vi "pump_main.vi"(8 "error in (no error)":errorcluster, 10 "input string":string, 11 "VISA resource name":refnum<visa-resource-name>) -> (0 "error out":errorcluster, 3 "VISA resource name out":refnum<visa-resource-name>)   [LabVIEW 2020]
uses:
  status/emergency stop.vi
panel:
  out "current time 2":timestamp
  out "current time":timestamp
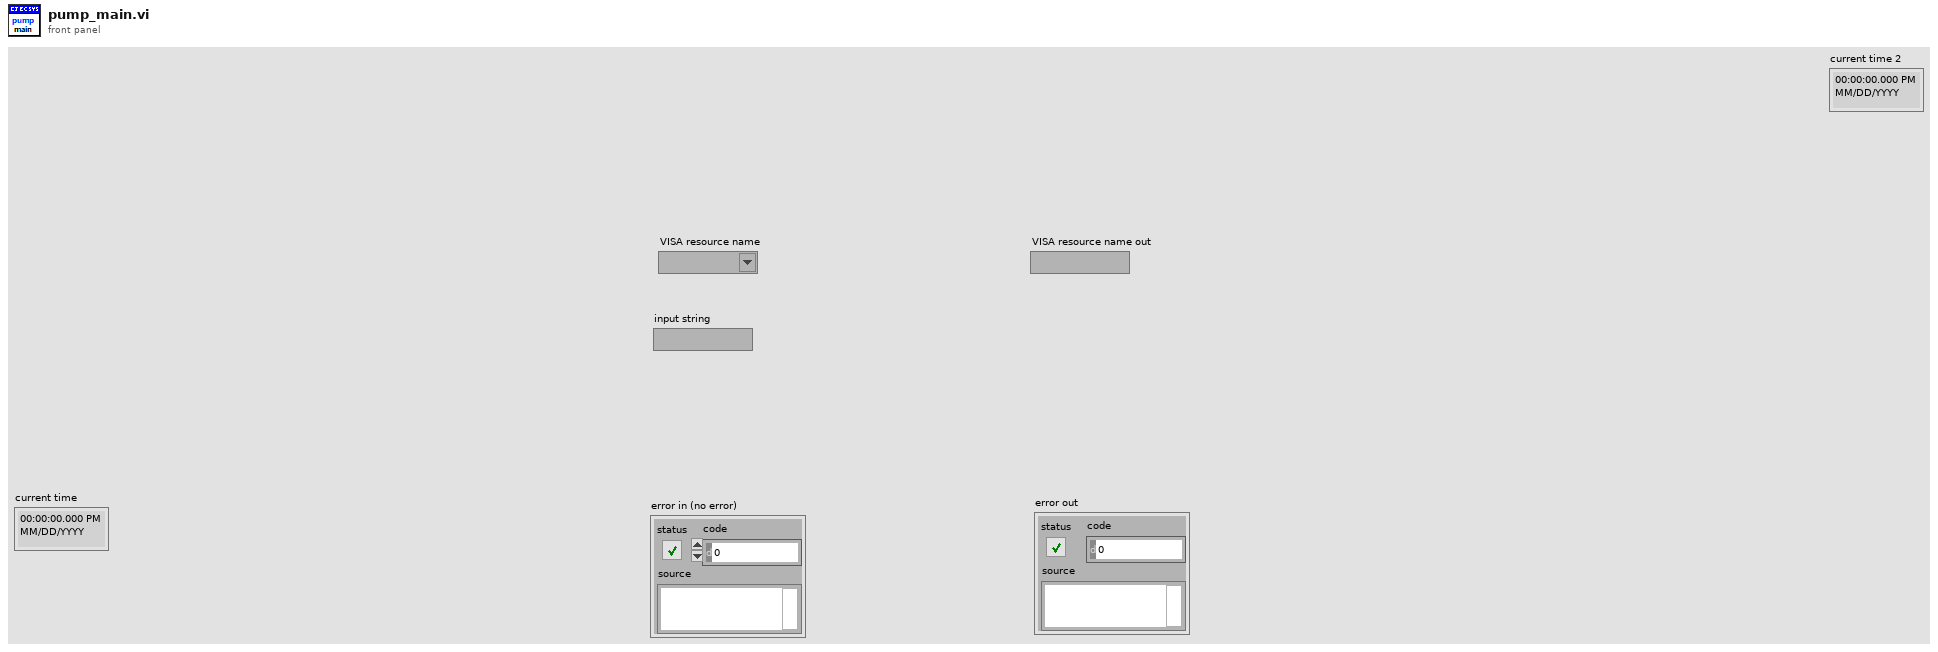
[diagram p1: front panel]
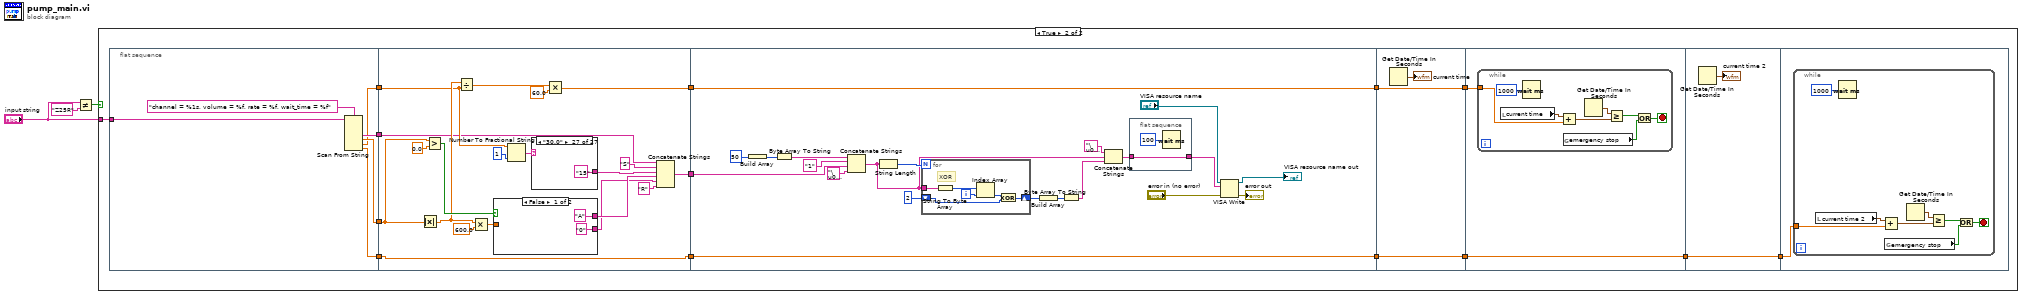
[diagram p0: block diagram]
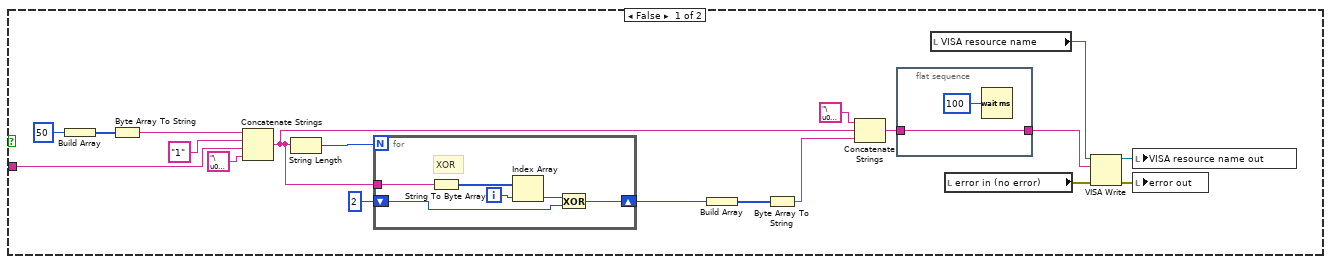
[diagram p2: hidden frame]
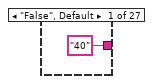
[diagram p3: hidden frame]
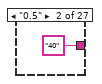
[diagram p4: hidden frame]
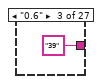
[diagram p5: hidden frame]
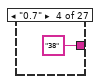
[diagram p6: hidden frame]
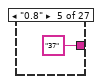
[diagram p7: hidden frame]
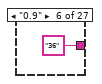
[diagram p8: hidden frame]
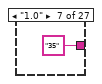
[diagram p9: hidden frame]
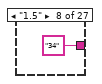
[diagram p10: hidden frame]
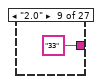
[diagram p11: hidden frame]
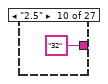
[diagram p12: hidden frame]
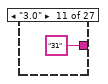
[diagram p13: hidden frame]
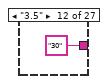
[diagram p14: hidden frame]
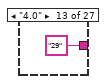
[diagram p15: hidden frame]
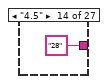
[diagram p16: hidden frame]
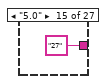
[diagram p17: hidden frame]
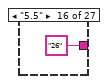
[diagram p18: hidden frame]
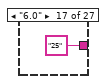
[diagram p19: hidden frame]
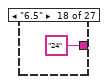
[diagram p20: hidden frame]
diagram:
  n1 = Not Equal?(x="input string", y="Z25R") -> (x != y?=w1:bool)
  n2 = case shown="True" w1 {
    tunnel: "input string" -> [w4 w31]
    frame False {
      n3 = Build Array(u8 50 ("y")) -> (w12:u8[])
      n4 = Byte Array To String(unsigned byte array=w12) -> (string=w10:string)
      n5 = Concatenate Strings(w10, "1" ("string"), w4, "\u0003" ("string")) -> (w16:string)
      n6 = String Length(string=w16) -> (length=w22:i32)
      n7 = for {
        N: w22 -> [_]
        tunnel: w16 -> [w30]
        shift-right: [w25] -> w20
        shift-left: u8 2 -> [w26]
        i -> [w28]
        # "XOR"
        n8 = String To Byte Array(string=w30) -> (unsigned byte array=w29:u8[])
        n9 = Index Array(array=w29, index=w28) -> (element=w27:u8)
        n10 = Exclusive Or(1:w26, 2:w27) -> (0:w25:u8)
      }
      n11 = Build Array(w20) -> (w19:u8[])
      n12 = Byte Array To String(unsigned byte array=w19) -> (string=w17:string)
      n13 = Concatenate Strings("\u0002" ("string"), w16, w17) -> (w15:string)
      n14 = flat-sequence {
        tunnel: [w24] -> w14
        tunnel: w15 -> [w24]
        frame #0 {
          n15 = Wait (ms)(milliseconds to wait=u32 100) -> ()  [unwired: 1 out]
        }
      }
      n16 = local read "VISA resource name"() -> (w8:refnum<visa-resource-name>)
      n17 = local read "error in (no error)"() -> (w7:errorcluster)
      n18 = VISA Write(VISA resource name=w8, write buffer=w14, error in (no error)=w7) -> (VISA resource name out=w6:refnum<visa-resource-name>, error out=w5:errorcluster)  [unwired: 1 out]
      n19 = local write "VISA resource name out"(w6) -> ()
      n20 = local write "error out"(w5) -> ()
    }
    frame True {
      n21 = flat-sequence {
        tunnel: [w49] -> w44
        tunnel: [w48] -> w43
        tunnel: [w47] -> w42
        tunnel: [w46] -> w41
        tunnel: w31 -> [w45]
        tunnel: [w66] -> w40
        tunnel: [w59] -> w39
        tunnel: w44 -> [w53]
        tunnel: w43 -> [w58]
        tunnel: w42 -> [w57]
        tunnel: w41 -> [w56]
        tunnel: [w56] -> w38
        tunnel: w40 -> [w109]
        tunnel: w39 -> [w104]
        tunnel: [w104] -> w37
        tunnel: w38 -> [w103]
        tunnel: [w103] -> w36
        tunnel: w37 -> [w133]
        tunnel: [w133] -> w35
        tunnel: [w132] -> w34
        tunnel: w36 -> [w132]
        tunnel: w35 -> [w136]
        tunnel: w34 -> [w135]
        tunnel: [w135] -> w33
        tunnel: w33 -> [w145]
        tunnel: [w145] -> w32
        tunnel: w32 -> [w147]
        frame #0 {
          n22 = Scan From String(format string="channel = %1s, volume = %f, rate = %f, wait_time = %f", input string=w45) -> (output 1=w49:string, output 2=w48:dbl, output 3=w47:dbl, output 4=w46:dbl)  [unwired: 6 in, 3 out]
        }
        frame #1 {
          n23 = Absolute Value(x=w58) -> (abs(x)=w62:dbl)
          n24 = Greater?(x=w58, y=0.0) -> (0:w69:bool)
          n25 = Divide(x=w62, y=w57) -> (x/y=w61:dbl)
          n26 = Multiply(x=w62, y=600.0) -> (x*y=w52:dbl)
          n27 = case shown="False" w69 {
            tunnel: ["A" ("channel") "P" ("channel")] -> w70
            tunnel: w52 -> [_ w101]
            tunnel: ["0" w100] -> w51
            frame False {
            }
            frame True {
              n28 = Number To Decimal String(number=w101) -> (decimal integer string=w100:string)  [unwired: 1 in]
            }
          }
          n29 = Number To Fractional String(number=w57, precision (6)=i16 1) -> (F-format string=w65:string)  [unwired: 2 in]
          n30 = case shown="\"30.0\"" w65 {
            tunnel: ["40" "40" "39" "38" "37" "36" "35" "34" "33" "32" "31" "30" "29" "28" "27" "26" "25" "24" "23" "22" "21" "20" "19" "18" "17" "16" "15"] -> w55
            frame "False", Default {
            }
            frame "0.5" {
            }
            frame "0.6" {
            }
            frame "0.7" {
            }
            frame "0.8" {
            }
            frame "0.9" {
            }
            frame "1.0" {
            }
            frame "1.5" {
            }
            frame "2.0" {
            }
            frame "2.5" {
            }
            frame "3.0" {
            }
            frame "3.5" {
            }
            frame "4.0" {
            }
            frame "4.5" {
            }
            frame "5.0" {
            }
            frame "5.5" {
            }
            frame "6.0" {
            }
            frame "6.5" {
            }
            frame "7.0" {
            }
            frame "7.5" {
            }
            frame "8.0" {
            }
            frame "8.5" {
            }
            frame "9.0" {
            }
            frame "9.5" {
            }
            frame "10.0" {
            }
            frame "20.0" {
            }
            frame "30.0" {
            }
          }
          n31 = Multiply(x=w61, y=60.0) -> (x*y=w59:dbl)
          n32 = Concatenate Strings(w53, "S" ("string"), w55, w70, w51, "R" ("string")) -> (w66:string)
        }
        frame #2 {
          n33 = Build Array(u8 50 ("y")) -> (w108:u8[])
          n34 = Byte Array To String(unsigned byte array=w108) -> (string=w106:string)
          n35 = Concatenate Strings(w106, "1" ("string"), w109, "\u0003" ("string")) -> (w117:string)
          n36 = String Length(string=w117) -> (length=w123:i32)
          n37 = for {
            N: w123 -> [_]
            tunnel: w117 -> [w131]
            shift-right: [w126] -> w121
            shift-left: u8 2 -> [w127]
            i -> [w129]
            # "XOR"
            n38 = String To Byte Array(string=w131) -> (unsigned byte array=w130:u8[])
            n39 = Index Array(array=w130, index=w129) -> (element=w128:u8)
            n40 = Exclusive Or(1:w127, 2:w128) -> (0:w126:u8)
          }
          n41 = Build Array(w121) -> (w120:u8[])
          n42 = Byte Array To String(unsigned byte array=w120) -> (string=w118:string)
          n43 = Concatenate Strings("\u0002" ("string"), w117, w118) -> (w114:string)
          n44 = flat-sequence {
            tunnel: [w125] -> w113
            tunnel: w114 -> [w125]
            frame #0 {
              n45 = Wait (ms)(milliseconds to wait=u32 100) -> ()  [unwired: 1 out]
            }
          }
          n46 = VISA Write(VISA resource name="VISA resource name", write buffer=w113, error in (no error)="error in (no error)") -> (VISA resource name out=→"VISA resource name out":refnum<visa-resource-name>, error out=→"error out":errorcluster)  [unwired: 1 out]
        }
        frame #3 {
          n47 = Get Date/Time In Seconds() -> (seconds since 1Jan1904=→"current time":timestamp)
        }
        frame #4 {
          n48 = while {
            tunnel: w136 -> [w138]
            stop <- w139 stop-if-true
            n49 = local read "current time"() -> (w143:timestamp)
            n50 = Wait (ms)(milliseconds to wait=u32 1000 ("millisecond timer value")) -> ()  [unwired: 1 out]
            n51 = Add(x=w143, y=w138) -> (x+y=w142:timestamp)
            n52 = global read "emergency stop.vi" "emergency stop"() -> (w137:bool)
            n53 = Get Date/Time In Seconds() -> (seconds since 1Jan1904=w141:timestamp)
            n54 = Greater Or Equal?(x=w141, y=w142) -> (x >= y?=w140:bool)
            n55 = Or(x=w140, y=w137) -> (x .or. y?=w139:bool)
          }
        }
        frame #5 {
          n56 = Get Date/Time In Seconds() -> (seconds since 1Jan1904=→"current time 2":timestamp)
        }
        frame #6 {
          n57 = while {
            tunnel: w147 -> [w149]
            stop <- w150 stop-if-true
            n58 = local read "current time 2"() -> (w154:timestamp)
            n59 = Wait (ms)(milliseconds to wait=u32 1000 ("millisecond timer value")) -> ()  [unwired: 1 out]
            n60 = Add(x=w154, y=w149) -> (x+y=w153:timestamp)
            n61 = global read "emergency stop.vi" "emergency stop"() -> (w148:bool)
            n62 = Get Date/Time In Seconds() -> (seconds since 1Jan1904=w152:timestamp)
            n63 = Greater Or Equal?(x=w152, y=w153) -> (x >= y?=w151:bool)
            n64 = Or(x=w151, y=w148) -> (x .or. y?=w150:bool)
          }
        }
      }
    }
  }
